vi "Query Analog Output Scaling.vi"(8 "error in (no error)":errorcluster, 11 "VISA resource name":refnum<visa-resource-name>) -> (0 "error out":errorcluster, 1 "Current Scaling (volts)":i32(ring)=5 items=["3"=3, "5"=5, "10"=10], 2 "Voltage Scaling (volts)":i32(ring)=5 items=["3"=3, "5"=5, "10"=10], 3 "VISA resource name out":refnum<visa-resource-name>)   [LabVIEW 2018, in "XP Power PLS600.lvlib"]
doc: "Queries the scaling level of the voltage and current analog output channels."
uses:
  XP Power PLS600.lvlib
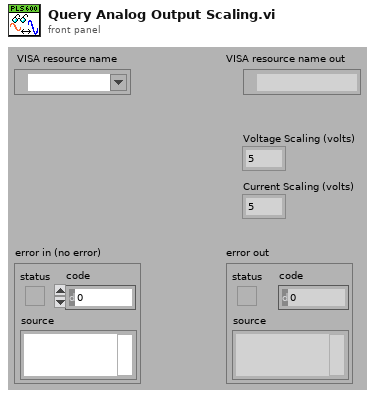
[diagram p1: front panel]
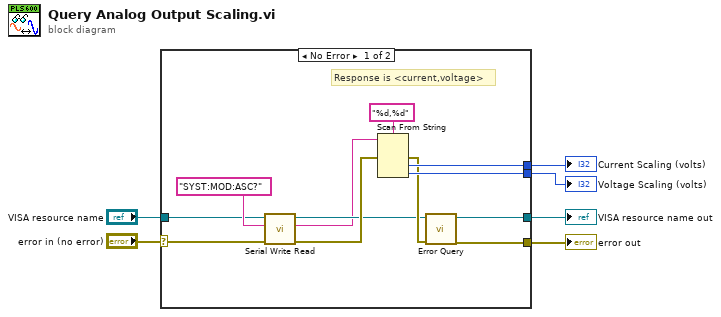
[diagram p0: block diagram]
diagram:
  n1 = case shown="No Error" "error in (no error)" {
    selector: "error in (no error)" -> [w7 w19]
    tunnel: [w18 w20] -> w6
    tunnel: [w17 w19] -> w5
    tunnel: [w15 _] -> w4
    tunnel: [w14 _] -> w3
    tunnel: "VISA resource name" -> [w8 w20]
    frame No Error {
      # "Response is <current,voltage>"
      n2 = call "Serial Write Read.vi"("error in (no error)"=w7, "Write Buffer"="SYST:MOD:ASC?", "VISA resource name"=w8) -> ("error out"=w12:errorcluster, "Read Buffer"=w10:string, "VISA resource name out"=w11:refnum<visa-resource-name>)  [unwired: 6 in]
      n3 = Scan From String(format string="%d,%d", input string=w10, error in=w12) -> (error out=w13:errorcluster, output 1=w15:i32, output 2=w14:i32)  [unwired: 3 in, 2 out]
      n4 = call "Error Query.vi"("error in (no error)"=w13, "VISA resource name"=w11) -> ("error out"=w17:errorcluster, "VISA resource name out"=w18:refnum<visa-resource-name>)  [unwired: 6 in, 2 out]
    }
    frame Error {
    }
  }
  "Voltage Scaling (volts)" <- w3
  "VISA resource name out" <- w6
  "error out" <- w5
  "Current Scaling (volts)" <- w4
